vi "panel_launch_subpanel_actor.vi"(8 "error in (no error)":errorcluster, 9 "Open Actor Core front panel? (F)":bool, 10 "nested_panel":refnum<class "panel.lvclass">, 11 "caller_panel":refnum<class "panel.lvclass">) -> (0 "error out":errorcluster, 1 "subpanel_reference":refnum<vi>, 2 "Nested Actor's Enqueuer":refnum<class "Message Enqueuer.lvclass">, 3 "Caller Actor out":refnum<class "panel.lvclass">, 4 "timed out?":bool)   [LabVIEW 2015, in "panel.lvclass"]
uses:
  panel.lvclass
  <vilib>/ActorFramework/Message Enqueuer/Message Enqueuer.lvclass
  <vilib>/ActorFramework/Actor/Actor.lvclass
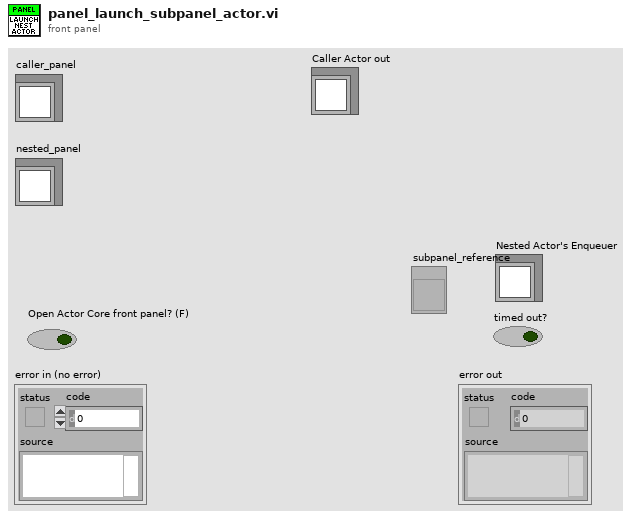
[diagram p1: front panel]
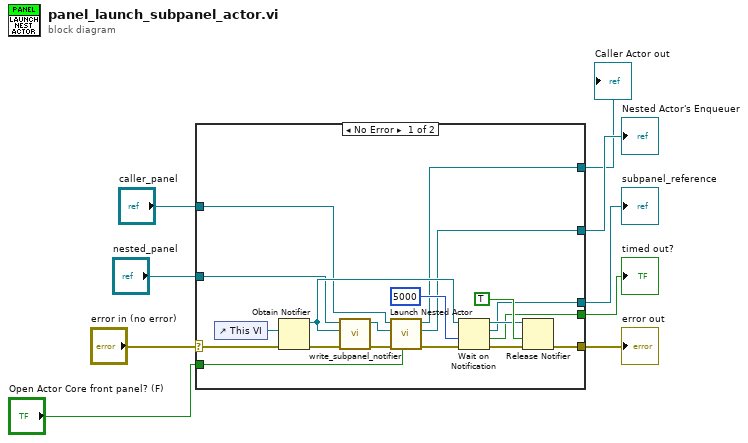
[diagram p0: block diagram]
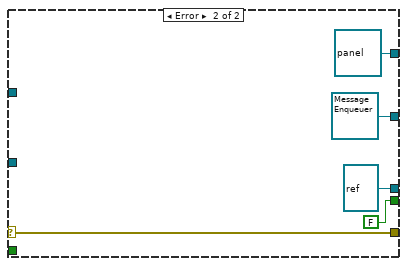
[diagram p2: hidden frame]
diagram:
  n1 = case shown="No Error" "error in (no error)" {
    selector: "error in (no error)" -> [w18 w33]
    tunnel: [w17 w33] -> w8
    tunnel: "caller_panel" -> [w16 _]
    tunnel: [w15 refnum<class "panel.lvclass"> refnum ("Caller Actor out")] -> w1
    tunnel: "nested_panel" -> [w14 _]
    tunnel: "Open Actor Core front panel? (F)" -> [w13 _]
    tunnel: [w12 FALSE ("timed out?")] -> w5
    tunnel: [w11 refnum<vi> refnum ("This VI")] -> w4
    tunnel: [w10 refnum<class "Message Enqueuer.lvclass"> refnum ("Nested Actor's Enqueuer")] -> w3
    frame No Error {
      n2 = control-ref of="This VI"() -> (w23:refnum<vi>)
      n3 = Obtain Notifier(notification data type=w23, error in (no error)=w18) -> (notifier out=w19:refnum<notifier>, error out=w22:errorcluster)  [unwired: 2 in, 1 out]
      n4 = call "write_subpanel_notifier.vi"("error in (no error)"=w22, "subpanel_notifier"=w19, "panel in"=w14) -> ("error out"=w21:errorcluster, "panel out"=w20:refnum<class "panel.lvclass">)  [unwired: 7 in]
      n5 = call <vilib>:"Launch Nested Actor.vi"("Open Actor Core front panel? (F)"=w13, "error in (no error)"=w21, "Nested Actor"=w20, "Caller Actor in"=w16) -> ("error out"=w24:errorcluster, "Nested Actor's Enqueuer"=w10:refnum<class "Message Enqueuer.lvclass">, "Caller Actor out"=w15:refnum<class "panel.lvclass">)  [unwired: 5 in]
      n6 = Wait on Notification(notifier=w19, timeout in ms (-1)=5000, error in (no error)=w24) -> (notifier out=w27:refnum<notifier>, notification=w11:refnum<vi>, timed out?=w12:bool, error out=w26:errorcluster)  [unwired: 1 in]
      n7 = Release Notifier(notifier=w27, force destroy? (F)=TRUE, error in (no error)=w26) -> (error out=w17:errorcluster)  [unwired: 2 out]
    }
    frame Error {
    }
  }
  "error out" <- w8
  "timed out?" <- w5
  "subpanel_reference" <- w4
  "Nested Actor's Enqueuer" <- w3
  "Caller Actor out" <- w1
